vi "distanceCalculator.vi"(9 "Limelight Version":enum16{"Limelight 2", "Limelight 1"}(ring), 11 "Target Width(px)":dbl) -> (2 "Distance From Target(Inches)":dbl)   [LabVIEW 2018]
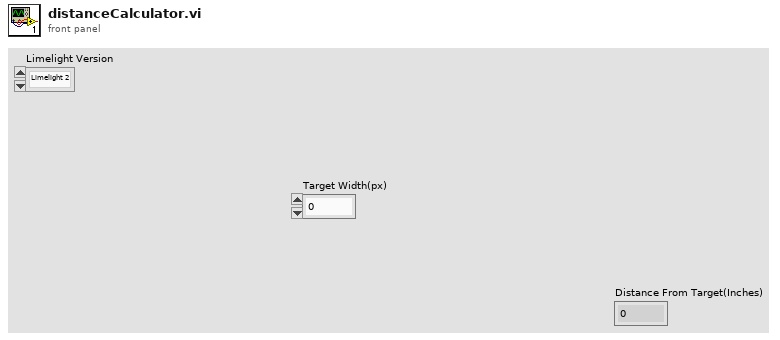
[diagram p1: front panel]
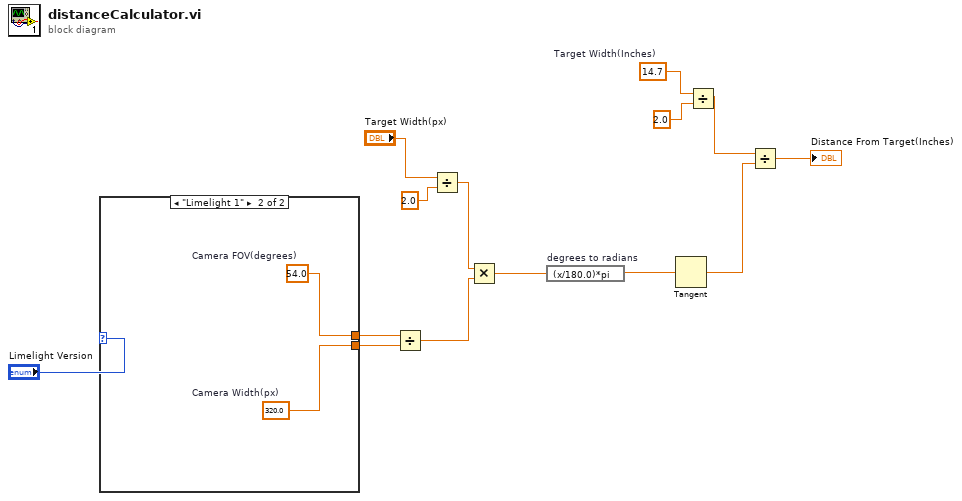
[diagram p0: block diagram]
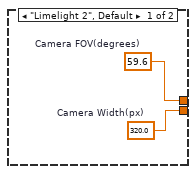
[diagram p2: hidden frame]
diagram:
  w5 = 14.7  # Target Width(Inches)
  n1 = case shown="\"Limelight 1\"" "Limelight Version" {
    tunnel: [w16 w18] -> w12
    tunnel: [w15 w17] -> w11
    frame "Limelight 2", Default {
      w15 = 320.0  # Camera Width(px)
      w16 = 59.6  # Camera FOV(degrees)
    }
    frame "Limelight 1" {
      w17 = 320.0  # Camera Width(px)
      w18 = 54.0  # Camera FOV(degrees)
    }
  }
  n2 = Divide(x=w12, y=w11) -> (x/y=w10:dbl)
  n3 = Divide(x="Target Width(px)", y=2.0) -> (x/y=w9:dbl)
  n4 = Multiply(x=w9, y=w10) -> (x*y=w3:dbl)
  n5 = expression code="(x/180.0)*pi" "degrees to radians"(w3) -> (w2:dbl)
  n6 = Tangent(1:w2) -> (0:w8:dbl)
  n7 = Divide(x=w5, y=2.0) -> (x/y=w6:dbl)
  n8 = Divide(x=w6, y=w8) -> (x/y=→"Distance From Target(Inches)":dbl)
